vi "读取电压.vi"(8 "错误输入（无错误）":errorcluster, 11 "VISA资源名称":refnum<visa-resource-name>) -> (0 "V2当前电压":dbl format="%_6g", 1 "V1当前电压":dbl format="%_6g", 2 "V2_Digital":string, 3 "V1_Digital":string)   [LabVIEW 2018]
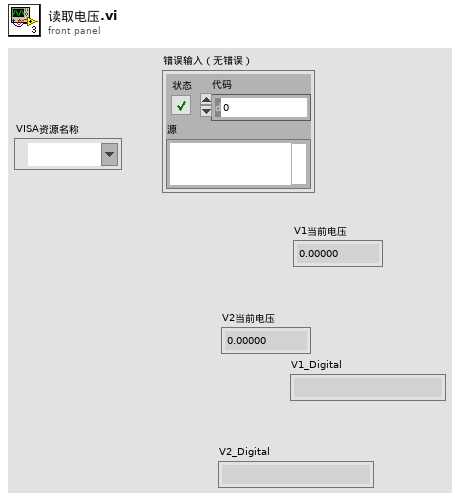
[diagram p1: front panel]
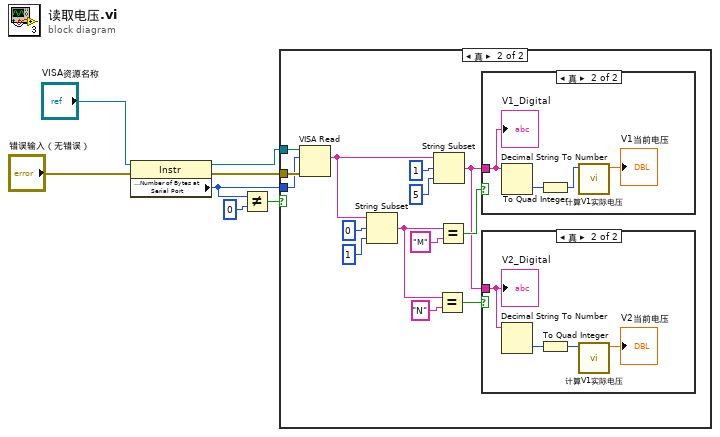
[diagram p0: block diagram]
diagram:
  n1 = property class="Instr"(reference="VISA资源名称", error in="错误输入（无错误）") -> (reference out=w6:refnum<visa-resource-name>, error out=w4:errorcluster, "Serial Settings:Number of Bytes at Serial Port"=w1:u32)
  n2 = Not Equal?(x=w1, y=0) -> (x != y?=w2:bool)
  n3 = case shown="真" w2 {
    tunnel: w6 -> [_ w21]
    tunnel: w4 -> [_ w20]
    tunnel: w1 -> [_ w8]
    frame False {
    }
    frame True {
      n4 = VISA Read(VISA resource name=w21, byte count=w8, error in (no error)=w20) -> (read buffer=w12:string)  [unwired: 3 out]
      n5 = String Subset(string=w12, offset (0)=0 ("偏移量(0)"), length (rest)=1 ("长度（剩余）")) -> (substring=w15:string)
      n6 = String Subset(string=w12, offset (0)=1, length (rest)=5) -> (substring=w9:string)
      n7 = Equal?(x=w15, y="N") -> (x = y?=w13:bool)
      n8 = Equal?(x=w15, y="M") -> (x = y?=w16:bool)
      n9 = case shown="真" w16 {
        tunnel: w9 -> [_ w26]
        frame False {
        }
        frame True {
          n10 = Decimal String To Number(string=w26) -> (number=w29:i32)  [unwired: 2 in, 1 out]
          n11 = To Quad Integer(1:w29) -> (0:w28:i64)
          n12 = call "计算V1实际电压.vi"("数值"=w28) -> ("x/y"=→"V1当前电压":dbl)  [unwired: 10 in]
          "V1_Digital" <- w26
        }
      }
      n13 = case shown="真" w13 {
        tunnel: w9 -> [_ w22]
        frame False {
        }
        frame True {
          n14 = Decimal String To Number(string=w22) -> (number=w25:i32)  [unwired: 2 in, 1 out]
          n15 = To Quad Integer(1:w25) -> (0:w24:i64)
          n16 = call "计算V1实际电压.vi"("数值"=w24) -> ("x/y"=→"V2当前电压":dbl)  [unwired: 10 in]
          "V2_Digital" <- w22
        }
      }
    }
  }
